vi "To XML.vi"(8 "error in (no error)":errorcluster, 9 "Parent":refnum<k20>, 10 "Document":refnum<k20>, 11 "Serializable in":refnum<class "Serializable.lvclass">) -> (0 "error out":errorcluster)   [LabVIEW 2017, in "Cobertura.lvlib" / "Serializable.lvclass"]
uses:
  Serializable.lvclass
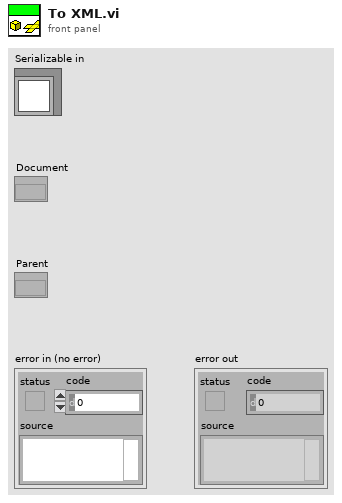
[diagram p1: front panel]
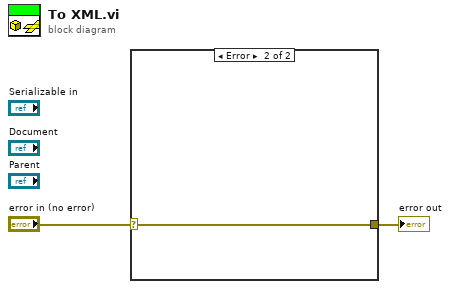
[diagram p0: block diagram]
diagram:
  n1 = case shown="Error" "error in (no error)" {
    selector: "error in (no error)" -> [w3 w4]
    tunnel: [w3 w4] -> w1
    frame No Error {
    }
    frame Error {
    }
  }
  "error out" <- w1
